vi "display.vi"(8 "error in (no error)":errorcluster, 11 "RubberDuck in":refnum<class "RubberDuck.lvclass">) -> (0 "error out":errorcluster, 2 "State":string, 3 "RubberDuck out":refnum<class "RubberDuck.lvclass">)   [LabVIEW 2013, in "RubberDuck.lvclass"]
uses:
  RubberDuck.lvclass
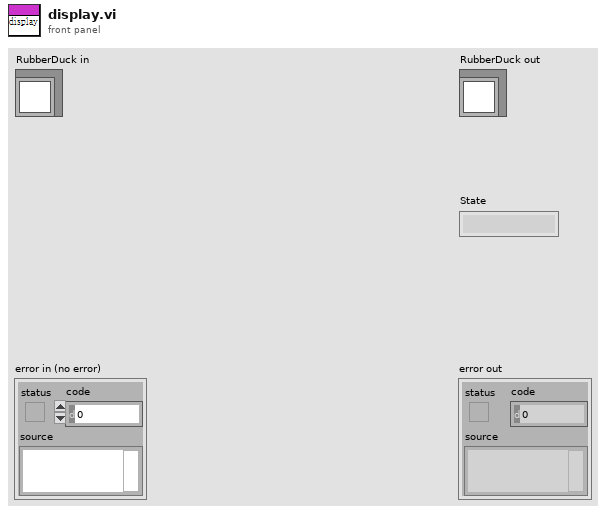
[diagram p1: front panel]
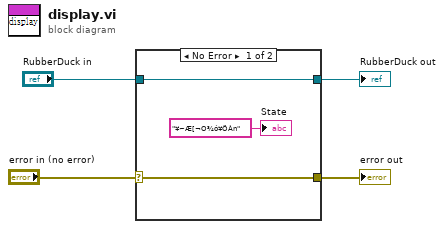
[diagram p0: block diagram]
diagram:
  n1 = case shown="No Error" "error in (no error)" {
    selector: "error in (no error)" -> [w7 w9]
    tunnel: [w7 w9] -> w3
    tunnel: [w5 w8] -> w2
    tunnel: "RubberDuck in" -> [w5 w8]
    frame No Error {
      "State" <- "¥~Æ[¬O¾ó¥ÖÀn" ("State")
    }
    frame Error {
    }
  }
  "error out" <- w3
  "RubberDuck out" <- w2
